vi "Stop Core.vi"(10 "final error code":i32, 11 "Actor Nest in":refnum<class "Actor Nest.lvclass">) -> (3 "Actor Nest out":refnum<class "Actor Nest.lvclass">)   [LabVIEW 2012, in "Actor Nest.lvlib" / "Actor Nest.lvclass"]
doc: "(<B>Filename</B>: Actor Framework.lvlib:Actor.lvclass:Stop Core.vi)\n\nDefines what the actor does before it stops. Use the <B>final error code</B> input to determine whether the actor shut down in response to an error.\n\nBy default, this method does nothing. A descendant class may override it to define behavior, such as shutting down any processes the actor initiated in its override of the Actor Core method."
uses:
  Actor Nest.lvclass
  Actor Nest.lvclass/Actor Nest.ctl
  <vilib>/ActorFramework/Actor/Actor.lvclass
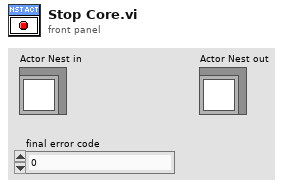
[diagram p1: front panel]
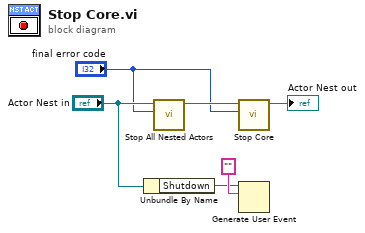
[diagram p0: block diagram]
diagram:
  n1 = Unbundle By Name("Actor Nest in") -> ("Shutdown"=w4:refnum<user-event>)
  n2 = call "Stop All Nested Actors.vi"("final error code"="final error code", "Actor Nest in"="Actor Nest in") -> ("Actor Nest out"=w2:refnum<class "Actor Nest.lvclass">)  [unwired: 8 in, 1 out]
  n3 = call-parent "Stop Core.vi"("final error code"="final error code", "Actor in"=w2) -> ("Actor out"=→"Actor Nest out":refnum<class "Actor Nest.lvclass">)  [unwired: 9 in]
  n4 = Generate User Event(user event=w4, event data cluster="" ("event data")) -> ()  [unwired: 1 in, 2 out]
